vi "Generate Password 32 characters.vi"(11 "error in (no error)":errorcluster) -> (6 "Password Byte [ ]":u8[](array[numeric]), 8 "Password string":string, 15 "error out":errorcluster)   [LabVIEW 2019]
doc: "Version 1.0\nDeveloped by Jean-Marc Simard\nCopyright © 2011, Exaprom Inc.\nAll rights reserved.\nLicense: BSD\n\nWith iTextSharp 4.1.6 (http://itextsharp.sourceforge.net)\nunder Mozilla Public License Version 1.1\n(http://www.mozilla.org/MPL/MPL-1.1.html)"
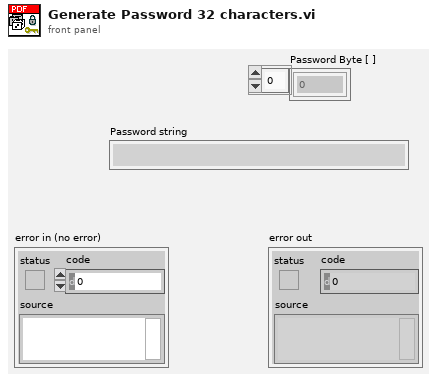
[diagram p1: front panel]
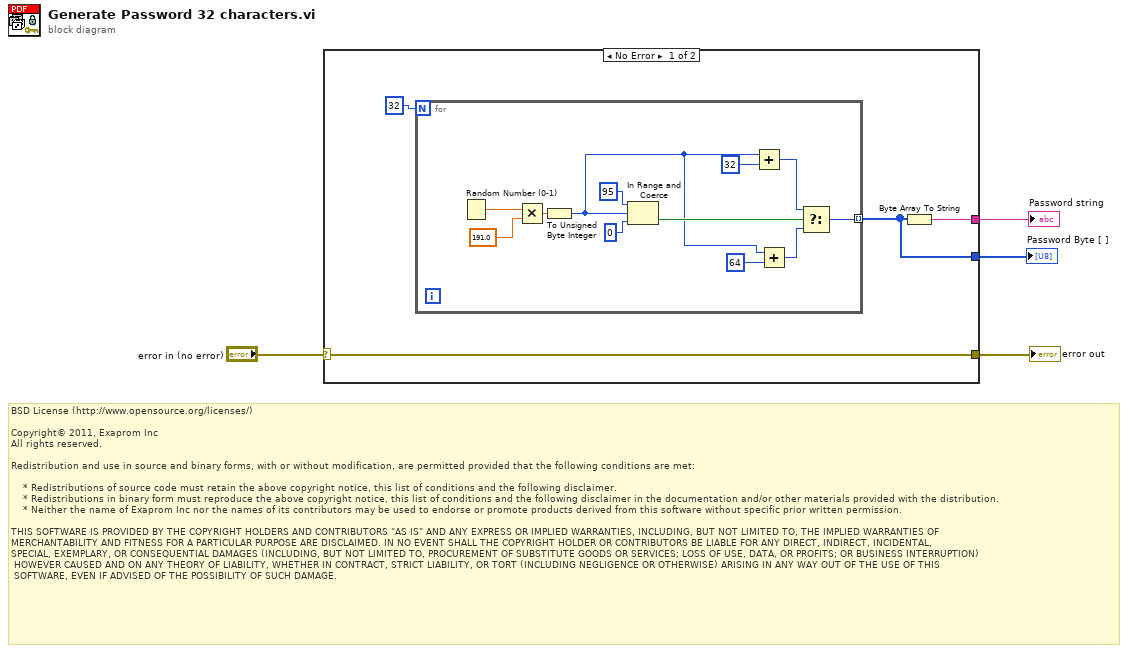
[diagram p0: block diagram]
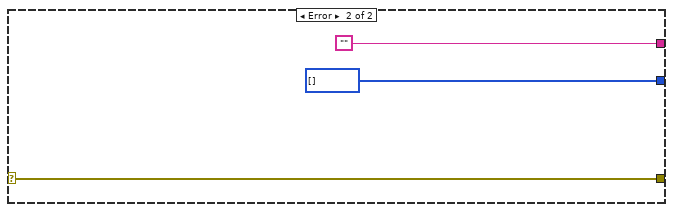
[diagram p2: hidden frame]
diagram:
  # "BSD License (http://www.opensource.org/licenses/)\n\nCopyright© 2011, Exaprom Inc\nAll rights reserved.\n\nRedistribution and use in source and binary forms, with or without modification, are permitted provided that the following conditions are met:\n\n    * Redistributions of source code must retain the above copyright notice, this list of conditions and the following disclaimer.\n    * Redistributions in binary form must reproduce the above copyright notice, this list of conditions and the following disclaimer in the documentation and/or other materials provided with the distribution.\n    * Neither the name of Exaprom Inc nor the names of its contributors may be used to endorse or promote products derived from this software without specific prior written permission.\n\nTHIS SOFTWARE IS PROVIDED BY THE COPYRIGHT HOLDERS AND CONTRIBUTORS \"AS IS\" AND ANY EXPRESS OR IMPLIED WARRANTIES, INCLUDING, BUT NOT LIMITED TO, THE IMPLIED WARRANTIES OF \nMERCHANTABILITY AND FITNESS FOR A PARTICULAR PURPOSE ARE DISCLAIMED. IN NO EVENT SHALL THE COPYRIGHT HOLDER OR CONTRIBUTORS BE LIABLE FOR ANY DIRECT, INDIRECT, INCIDENTAL,\nSPECIAL, EXEMPLARY, OR CONSEQUENTIAL DAMAGES (INCLUDING, BUT NOT LIMITED TO, PROCUREMENT OF SUBSTITUTE GOODS OR SERVICES; LOSS OF USE, DATA, OR PROFITS; OR BUSINESS INTERRUPTION)\n HOWEVER CAUSED AND ON ANY THEORY OF LIABILITY, WHETHER IN CONTRACT, STRICT LIABILITY, OR TORT (INCLUDING NEGLIGENCE OR OTHERWISE) ARISING IN ANY WAY OUT OF THE USE OF THIS\n SOFTWARE, EVEN IF ADVISED OF THE POSSIBILITY OF SUCH DAMAGE."
  n1 = case shown="No Error" "error in (no error)" {
    selector: "error in (no error)" -> [w8 w23]
    tunnel: [w8 w23] -> w4
    tunnel: [w6 u8[] []] -> w2
    tunnel: [w5 ""] -> w1
    frame No Error {
      n2 = for {
        N: 32 -> [_]
        tunnel: [w9] -> w6 mode=indexing
        n3 = Random Number (0-1)() -> (number: 0 to 1=w20:dbl)
        n4 = Multiply(x=w20, y=191.0) -> (x*y=w18:dbl)
        n5 = To Unsigned Byte Integer(number=w18) -> (unsigned 8bit integer=w10:u8)
        n6 = In Range and Coerce(upper limit=u8 95, x=w10, lower limit=u8 0) -> (In Range?=w15:bool)  [unwired: 1 out]
        n7 = Add(x=w10, y=u8 32) -> (x+y=w13:u8)
        n8 = Add(x=w10, y=u8 64) -> (x+y=w11:u8)
        n9 = Select(t=w13, s=w15, f=w11) -> (s? t:f=w9:u8)
      }
      n10 = Byte Array To String(unsigned byte array=w6) -> (string=w5:string)
    }
    frame Error {
    }
  }
  "error out" <- w4
  "Password Byte [ ]" <- w2
  "Password string" <- w1
